vi "Retrieve Actors.vi"(8 "error in (no error)":errorcluster, 11 "INI Store in":refnum<class "INI Store.lvclass">) -> (0 "error out":errorcluster, 1 "Actor Paths":path[](array[path]), 2 "Actors":string[](array[string]), 3 "INI Store out":refnum<class "INI Store.lvclass">)   [LabVIEW 2020, in "Add Actor.lvlib" / "INI Store.lvclass"]
uses:
  INI Store.lvclass
  <resource>/dialog/lvconfig.llb/LV Config Read String.vi
  <resource>/dialog/lvconfig.llb/LV Config Read Pathlist.vi
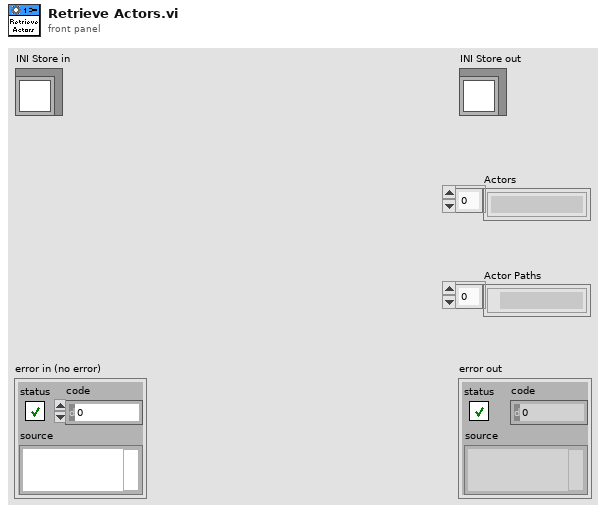
[diagram p1: front panel]
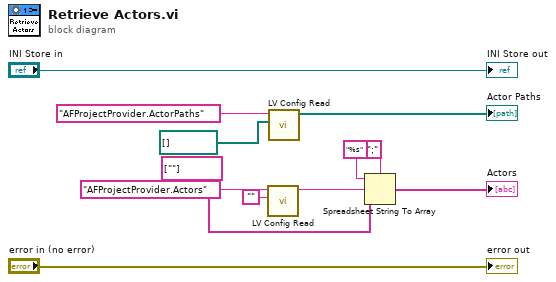
[diagram p0: block diagram]
diagram:
  n1 = call-poly <resource>:"LV Config Read.vi"("default value"="", "key"="AFProjectProvider.Actors") -> ("value"=w5:string)  [unwired: 3 in, 2 out]
  n2 = call-poly <resource>:"LV Config Read.vi"("default value"=path[] [] ("path"), "key"="AFProjectProvider.ActorPaths") -> ("value"=→"Actor Paths":path[])  [unwired: 3 in, 2 out]
  n3 = Spreadsheet String To Array(delimiter (Tab)=";", format string="%s", spreadsheet string=w5, array type (2D Dbl)=string[] [""]) -> (array=→"Actors":string[])
  "error out" <- "error in (no error)"
  "INI Store out" <- "INI Store in"
